vi "SbigQueryTemp.vi"(7 "SbigReference":T1, 9 "error in (no error)":errorcluster) -> (0 "Temperature Info":T2 {"Cooling %" format="%.2f"; "T Ambient" format="%.1f"; "T CCD" format="%.1f"; "T Setpoint" format="%.1f"}, 6 "error out":errorcluster)   [LabVIEW 2009]
uses:
  Controls/SbigReference.ctl
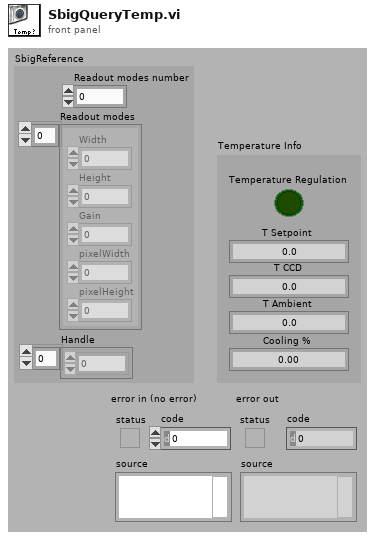
[diagram p1: front panel]
types:
  T1 = typedef "SbigReference.ctl" = cluster{"Readout modes number":u16, "Readout modes":cluster{"Width":u16, "Height":u16, "Gain":dbl, "pixelWidth":dbl, "pixelHeight":dbl}[], "Handle":u16[]}
  T2 = cluster{"Temperature Regulation":bool, "T Setpoint":dbl, "T CCD":dbl, "T Ambient":dbl, "Cooling %":dbl}
  T3 = enum16{"0-NoCommand", "1-StartExposure", "2-EndExposure", "3-ReadoutLine", "4-DumpLines", "5-SetTemperatureRegulation", "6-QueryTemperatureStatus", "7-ActivateRelay", "8-PulseOut", "9-EstablishLink", "10-GetDriverInfo", "11-GetCCDInfo", "12-QueryCommandStatus", "13-MiscellaneousControl", "14-ReadSubstractLine", "15-UpdateClock", "16-ReadOffset", "17-OpenDriver", "18-CloseDriver", "19-TXSerialBytes", "20-GetSerialStatus", "21-AOTipTilt", "22-AOSetFocus", "23-AODelay", "24-GetTurboStatus", "25-EndReadout", "26-GetUSTimer", "27-OpenDevice", "28-CloseDevice", "29-SetIRQL", "30-GetIRQL", "31-GetLine", "32-GetLinkStatus", "33-GetDriverHandle", "34-SetDriverHandle", "35-StartReadout", "36-GetErrorString", "37-SetDriverControl", "38-GetDriverControl", "39-USBADControl", "40-QueryUSB", "41-GetPentiumCycleCount", "42-RWUSBI2C", "43-CFW"}
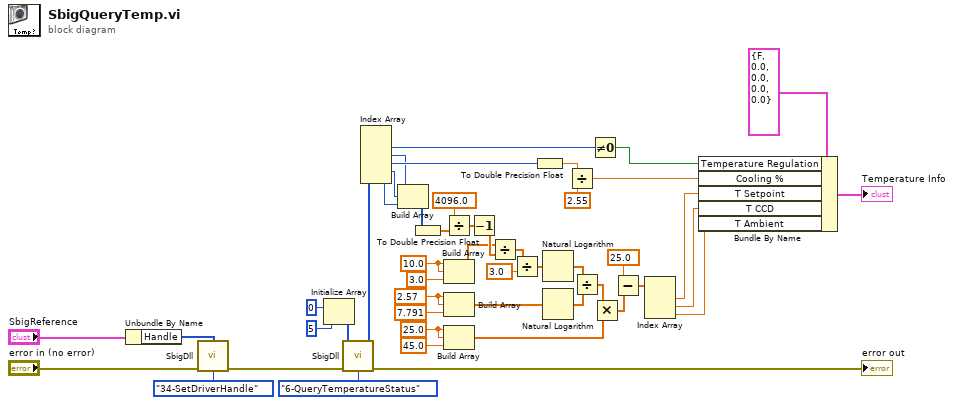
[diagram p0: block diagram]
diagram:
  w36 = 25.0
  w38 = 10.0
  w40 = 2.57
  n1 = Unbundle By Name("SbigReference") -> ("Handle"=w1:u16[])
  n2 = call "SbigDll.vi"("error in (no error)"="error in (no error)", "Command"=T3."34-SetDriverHandle", "Parameters"=w1) -> ("error out"=w11:errorcluster)  [unwired: 1 in, 3 out]
  n3 = Initialize Array(u16 0 ("Elément d'entrée"), 5 ("Taille de la dimension")) -> (w10:u16[])
  n4 = call "SbigDll.vi"("error in (no error)"=w11, "Command"=T3."6-QueryTemperatureStatus", "Results In"=w10) -> ("error out"=→"error out":errorcluster, "Results Out"=w15:u16[])  [unwired: 1 in, 2 out]
  n5 = Index Array(array=w15) -> (element #1=w46:u16, element #2=w43:u16, element #3=w45:u16, element #4=w42:u16, element #5=w41:u16)  [unwired: 5 in]
  n6 = Build Array(w43, w42, w41) -> (w34:u16[])
  n7 = To Double Precision Float(number=w34) -> (double precision float=w33:dbl[])
  n8 = Divide(x=4096.0, y=w33) -> (x/y=w31:dbl[])
  n9 = Build Array(w38, w38, 3.0 ("Elément d'entrée")) -> (w26:dbl[])
  n10 = Build Array(w40, w40, 7.791 ("Elément d'entrée")) -> (w25:dbl[])
  n11 = Build Array(w36, w36, 45.0 ("Elément d'entrée")) -> (w21:dbl[])
  n12 = Decrement(x=w31) -> (x-1=w30:dbl[])
  n13 = Divide(x=w26, y=w30) -> (x/y=w29:dbl[])
  n14 = Divide(x=w29, y=3.0) -> (x/y=w27:dbl[])
  n15 = To Double Precision Float(number=w45) -> (double precision float=w17:dbl)
  n16 = Natural Logarithm(1:w27) -> (0:w24:dbl[])
  n17 = Natural Logarithm(1:w25) -> (0:w23:dbl[])
  n18 = Divide(x=w17, y=2.55) -> (x/y=w6:dbl)
  n19 = Divide(x=w24, y=w23) -> (x/y=w22:dbl[])
  n20 = Not Equal To 0?(x=w46) -> (x != 0?=w7:bool)
  n21 = Multiply(x=w22, y=w21) -> (x*y=w20:dbl[])
  n22 = Subtract(x=25.0, y=w20) -> (x-y=w18:dbl[])
  n23 = Index Array(array=w18) -> (element #1=w5:dbl, element #2=w4:dbl, element #3=w3:dbl)  [unwired: 3 in]
  n24 = Bundle By Name(cluster=T2 {"Temperature Regulation"=FALSE, "T Setpoint"=0.0, "T CCD"=0.0, "T Ambient"=0.0, "Cooling %"=0.0} ("Temperature Info"), "Temperature Regulation"=w7, "Cooling %"=w6, "T Setpoint"=w5, "T CCD"=w4, "T Ambient"=w3) -> (→"Temperature Info":T2)
